vi "Execution Profiler View.vi"(8 "error in (no error)":errorcluster, 11 "Execution Profiler Result View":refnum<class "Execution Profiler Result View.lvclass">) -> (0 "error out":errorcluster)   [LabVIEW 2020, in "Execution Profiler.lvlib" / "Execution Profiler Result View.lvclass"]
uses:
  Execution Profiler Result View/Execution Profiler Result View.lvclass
  Execution Profiler Result View/Execution Profiler Result View.lvclass/Execution Profiler Result View.ctl
panel:
  in  "Method Test Times":i32(listbox)
  out "Histogram":cluster{"X":dbl, "Y":dbl}[](graph)
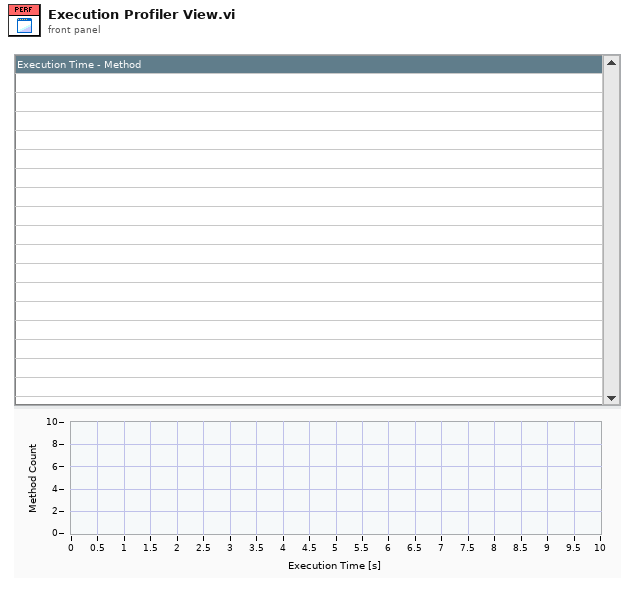
[diagram p1: front panel]
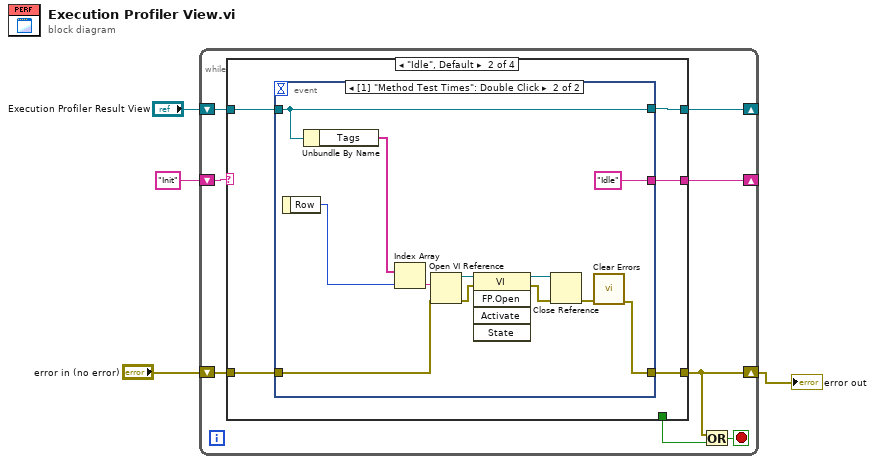
[diagram p0: block diagram]
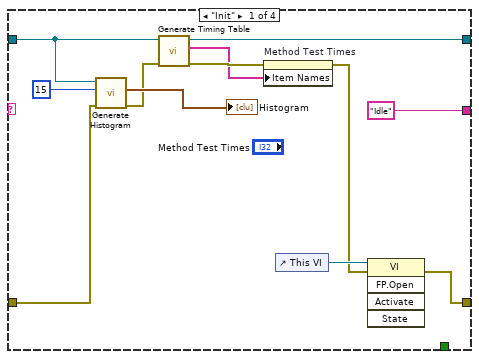
[diagram p2: hidden frame]
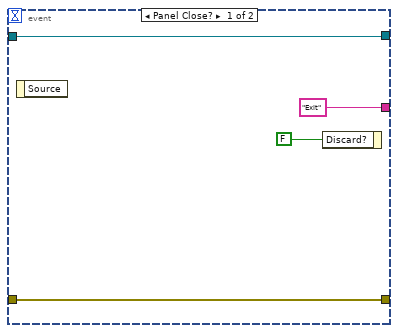
[diagram p3: hidden frame]
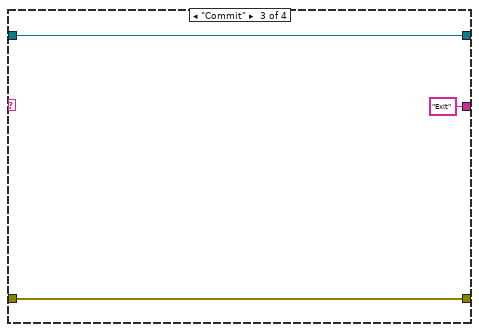
[diagram p4: hidden frame]
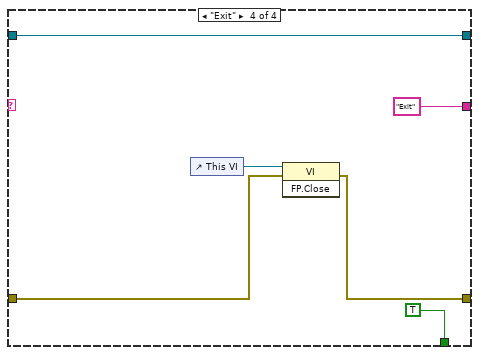
[diagram p5: hidden frame]
diagram:
  n1 = while {
    shift-right: [w9] -> _
    shift-left: "Execution Profiler Result View" -> [w10]
    shift-right: [w5] -> w2
    shift-left: "error in (no error)" -> [w11]
    shift-right: [w8] -> _
    shift-left: "Init" -> [w12]
    stop <- w6 stop-if-true
    n2 = case shown="\"Idle\", Default" w12 {
      tunnel: [w19 w29 w48 w50] -> w5
      tunnel: w11 -> [w22 w28 w48 w49]
      tunnel: w10 -> [w13 w27 w47 w54]
      tunnel: [w18 w26 w47 w54] -> w9
      tunnel: ["Idle" w25 "Exit" "Exit"] -> w8
      tunnel: [_ _ _ TRUE] -> w7
      frame "Init" {
        n3 = call "Generate Histogram.vi"("error in (no error)"=w22, "Interval Scaling"=u8 15 ("Number of intervals"), "View In"=w13) -> ("error out"=w17:errorcluster, "Histogram"=→"Histogram":cluster{dbl, dbl}[])  [unwired: 7 in]
        n4 = call "Generate Timing Table.vi"("error in (no error)"=w17, "Performance Analyzer In"=w13) -> ("error out"=w16:errorcluster, "Timing List"=w14:string[], "Performance Analyzer Out"=w18:refnum<class "Execution Profiler Result View.lvclass">)  [unwired: 7 in]
        n5 = property on="Method Test Times" class="LstBox (strict)"(error in=w16, "Item Names"=w14) -> (error out=w15:errorcluster)  [unwired: 1 in, 1 out]
        n6 = control-ref of="This VI"() -> (w20:refnum<vi>)
        n7 = invoke class="VI" method="FP.Open"(reference=w20, error in=w15) -> (error out=w19:errorcluster)  [unwired: 3 in, 4 out]
      }
      frame "Idle", Default {
        n8 = event shown="[1] \"Method Test Times\": Double Click" {
          selector: _ -> [_ _]
          dyn-events: _ -> [_ _]
          timeout: _ -> [_ _]
          tunnel: [w33 w34] -> w29
          tunnel: w28 -> [w33 w36]
          tunnel: w27 -> [w32 w43]
          tunnel: [w32 w43] -> w26
          tunnel: ["Exit" "Idle"] -> w25
          event Panel Close? {
            n9 = event-data() -> ()  [unwired: 1 in, 1 out]
            n10 = event-data("Discard?"=FALSE) -> ()  [unwired: 1 in, 1 out]
          }
          event "Method Test Times": Double Click {
            n11 = event-data() -> ("Row"=w44:i32)  [unwired: 1 in]
            n12 = Unbundle By Name(w43) -> ("Tags"=w42:string[])
            n13 = Index Array(array=w42, index=w44) -> (element=w41:string)
            n14 = Open VI Reference(vi path=w41, error in (no error)=w36) -> (vi reference=w40:refnum<vi>, error out=w37:errorcluster)  [unwired: 4 in]
            n15 = invoke class="VI" method="FP.Open"(reference=w40, error in=w37) -> (reference out=w39:refnum<vi>, error out=w38:errorcluster)  [unwired: 3 in, 3 out]
            n16 = Close Reference(reference=w39, error in (no error)=w38) -> (error out=w35:errorcluster)
            n17 = call <vilib>:"Clear Errors.vi"("error in (no error)"=w35) -> ("error out"=w34:errorcluster)  [unwired: 5 in, 1 out]
          }
        }
      }
      frame "Commit" {
      }
      frame "Exit" {
        n18 = control-ref of="This VI"() -> (w51:refnum<vi>)
        n19 = invoke class="VI" method="FP.Close"(reference=w51, error in=w49) -> (error out=w50:errorcluster)  [unwired: 1 in, 2 out]
      }
    }
    n20 = Or(x=w5, y=w7) -> (x .or. y?=w6:bool)
  }
  "error out" <- w2
